vi "Get Data Log File Settings.vi"(8 "error in (no error)":errorcluster, 11 "File Ref In":T1 format="%.0x") -> (0 "error out":errorcluster, 1 "Timestamp":bool, 2 "File Path":path, 3 "File Ref Out":T1 format="%.0x", 5 "Name":string)   [LabVIEW 2019, in "Telemetry System Explorer.lvlib"]
uses:
  Telemetry System Explorer.lvlib
  <vilib>/NI VeriStand/Custom Device API/Custom Device Item Ref.ctl
  Shared/Constants.vi
  <vilib>/NI VeriStand/Custom Device API/Get Item Property (String Array).vi
  <vilib>/NI VeriStand/Custom Device API/Get Item Property (Boolean).vi
  <vilib>/NI VeriStand/Custom Device API/Custom Device API.lvlib
  Shared/Telemetry Shared.lvlib
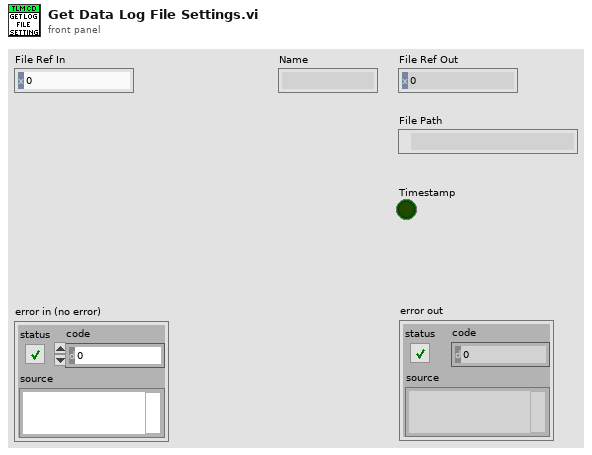
[diagram p1: front panel]
types:
  T1 = typedef "Custom Device API.lvlib/Custom Device Item Ref.ctl" = u64
  T2 = typedef "Custom Device API.lvlib/Custom Device Item Info.ctl" = cluster{"Name":string, "Is Channel":bool, "GUID":string, "Is Waveform":bool}
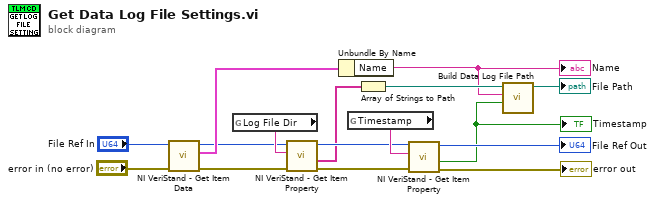
[diagram p0: block diagram]
diagram:
  n1 = call <vilib>:"NI VeriStand - Get Item Data.vi"("error in (no error)"="error in (no error)", "Item Ref in"="File Ref In") -> ("error out"=w13:errorcluster, "Item Info"=w14:T2, "Item Ref out"=w11:T1)  [unwired: 7 out]
  n2 = global read "Constants.vi" "Log File Dir"() -> (w12:string)
  n3 = call-poly <vilib>:"NI VeriStand - Get Item Property.vi"("error in (no error)"=w13, "Property Name"=w12, "Item Ref in"=w11) -> ("error out"=w8:errorcluster, "Value"=w6:string[], "Item Ref out"=w9:T1)  [unwired: 1 in, 5 out]
  n4 = Unbundle By Name(w14) -> ("Name"=w5:string)
  "Name" <- w5
  n5 = global read "Constants.vi" "Timestamp"() -> (w10:string)
  n6 = Array of Strings to Path(0:w6) -> (2:w7:path)  [unwired: 1 in]
  n7 = call-poly <vilib>:"NI VeriStand - Get Item Property.vi"("error in (no error)"=w8, "Property Name"=w10, "Item Ref in"=w9) -> ("error out"=→"error out":errorcluster, "Value"=w1:bool, "Item Ref out"=→"File Ref Out":T1)  [unwired: 1 in, 5 out]
  "Timestamp" <- w1
  n8 = call "Build Data Log File Path.vi"("Timestamp"=w1, "Name"=w5, "Log File Directory"=w7) -> ("appended path"=→"File Path":path)  [unwired: 7 in, 1 out]
